vi "NUMBER_PAD.vi"(0 "number (in)":i32) -> (4 "number (out)":i32)   [LabVIEW 2022 SP3]
panel:
  in  "Tab Control":enum32{"Page 1", "Page 2"}(tab)
  in  "Cancel":bool
  in  "Enter":bool
  in  "Clear":bool
  in  "0":bool
  in  "9":bool
  in  "8":bool
  in  "7":bool
  in  "6":bool
  in  "5":bool
  in  "4":bool
  in  "3":bool
  in  "2":bool
  in  "1":bool
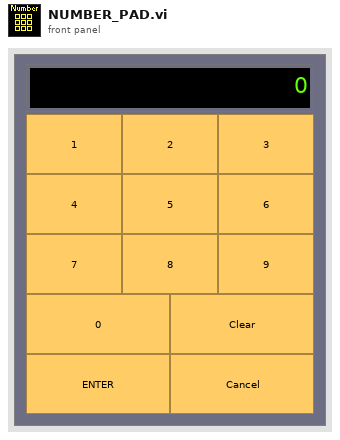
[diagram p1: front panel]
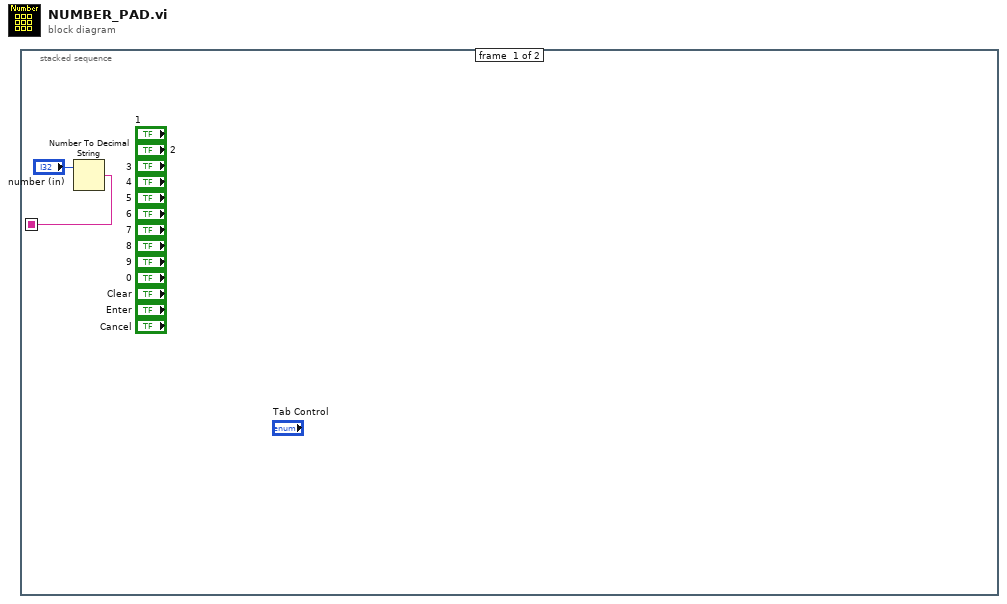
[diagram p0: block diagram]
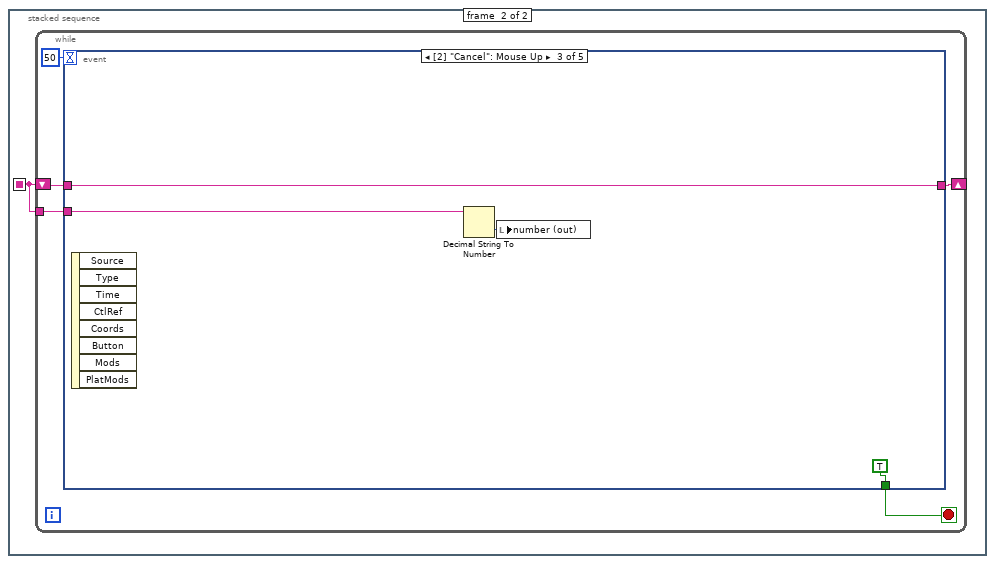
[diagram p2: hidden frame]
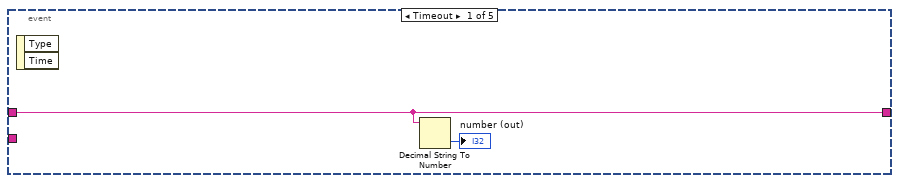
[diagram p3: hidden frame]
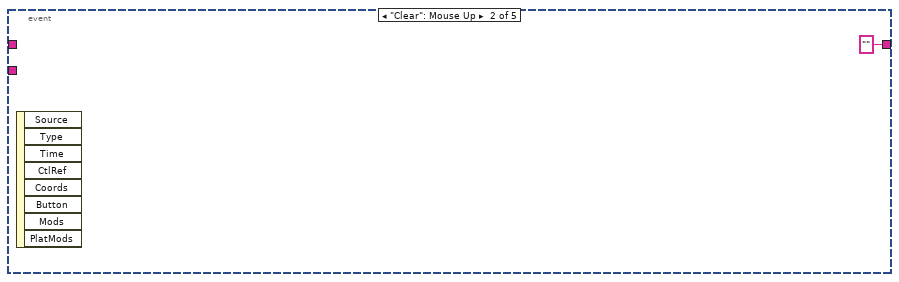
[diagram p4: hidden frame]
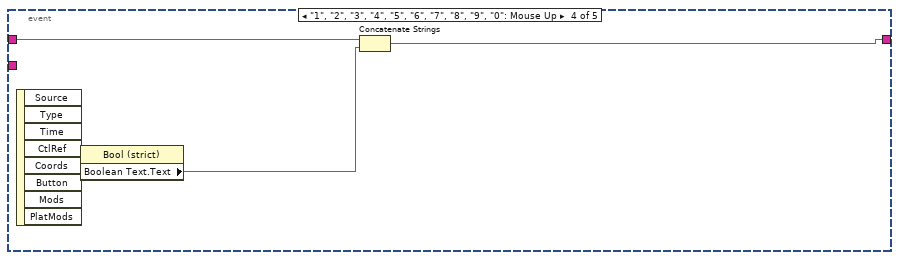
[diagram p5: hidden frame]
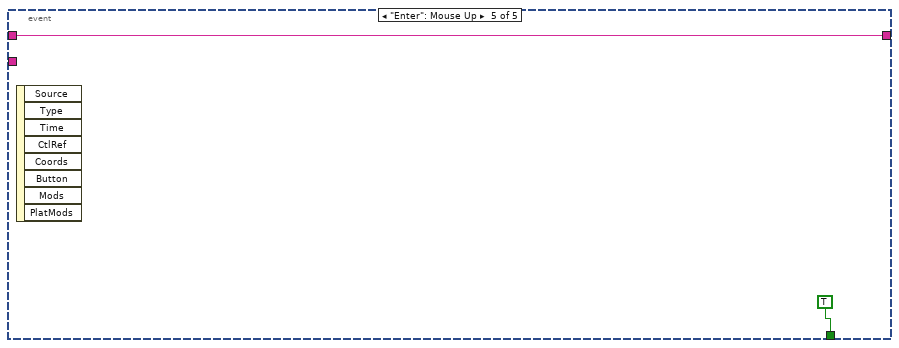
[diagram p6: hidden frame]
diagram:
  n1 = stacked-sequence {
    seq-local: [w1 _] -> [_ w3]
    frame #0 {
      n2 = Number To Decimal String(number="number (in)") -> (decimal integer string=w1:string)  [unwired: 1 in]
    }
    frame #1 {
      n3 = while {
        shift-right: [w7] -> _
        shift-left: w3 -> [w8]
        tunnel: w3 -> [w4]
        stop <- w6 stop-if-true
        n4 = event shown="[2] \"Cancel\": Mouse Up" {
          selector: _ -> [_ _ _ _ _]
          dyn-events: _ -> [_ _ _ _ _]
          timeout: 50 -> [_ _ _ _ _]
          tunnel: w8 -> [w10 _ w13 w19 w20]
          tunnel: [w10 "" w13 w18 w20] -> w7
          tunnel: [_ _ TRUE _ TRUE] -> w6
          tunnel: w4 -> [_ _ w12 _ _]
          event Timeout {
            n5 = event-data() -> ()  [unwired: 1 in, 2 out]
            n6 = Decimal String To Number(string=w10) -> (number=→"number (out)":i32)  [unwired: 2 in, 1 out]
          }
          event "Clear": Mouse Up {
            n7 = event-data() -> ()  [unwired: 1 in, 8 out]
          }
          event "Cancel": Mouse Up {
            n8 = event-data() -> ()  [unwired: 1 in, 8 out]
            n9 = Decimal String To Number(string=w12) -> (number=w14:i32)  [unwired: 2 in, 1 out]
            n10 = local write "number (out)"(w14) -> ()
          }
          event "1", "2", "3", "4", "5", "6", "7", "8", "9", "0": Mouse Up {
            n11 = event-data() -> ("CtlRef"=w17:refnum<vi>)  [unwired: 1 in, 7 out]
            n12 = property class="Bool (strict)"(reference=w17) -> ("Boolean Text.Text"=w16:string)  [unwired: 1 in, 2 out]
            n13 = Concatenate Strings(w19, w16) -> (w18:string)
          }
          event "Enter": Mouse Up {
            n14 = event-data() -> ()  [unwired: 1 in, 8 out]
          }
        }
      }
    }
  }
